vi "Run EU and SR Factories.vi"(8 "error in":errorcluster, 11 "custom device":T1 format="%.0x") -> (0 "error out":errorcluster, 1 "tx execution unit":refnum<class "Tx Execution Unit.lvclass">, 2 "rx execution unit":refnum<class "Rx Execution Unit.lvclass">, 3 "custom device out":T1 format="%.0x", 4 "shared resources":refnum<class "Shared Resources.lvclass">)   [LabVIEW 2020, in "Create Execution Unit.lvclass"]
uses:
  Create Execution Unit.lvclass
  <vilib>/NI VeriStand/Custom Device API/Custom Device Item Ref.ctl
  Engine/Implementation/Tx Execution Unit/Tx Execution Unit.lvclass
  Engine/Implementation/Rx Execution Unit/Rx Execution Unit.lvclass
  Engine/Interfaces/Shared Resources/Shared Resources.lvclass
  Engine/Implementation/Execution Unit Factory/Execution Unit Factory.lvclass
  Engine/Implementation/Shared Resources Factory/Shared Resources Factory.lvclass
  <vilib>/NI VeriStand/Custom Device API/Custom Device API.lvlib
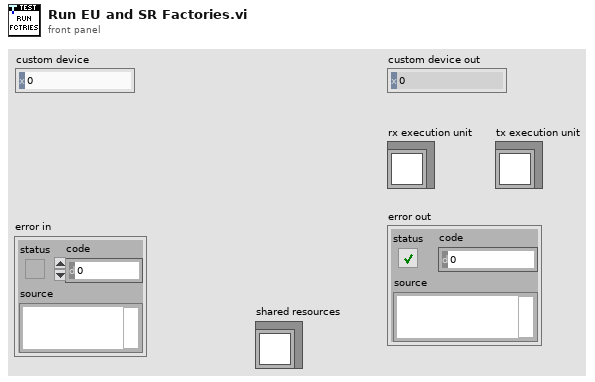
[diagram p1: front panel]
types:
  T1 = typedef "Custom Device API.lvlib/Custom Device Item Ref.ctl" = u64
  T2 = typedef "AIM MIL-STD-1553 Engine.lvlib/Interfaces.lvlib/Execution Unit Information.ctl" = cluster{"Execution Unit":refnum<class "Execution Unit.lvclass">, "Incoming Channels":T1[], "Outgoing Channels":T1[], "ReadWrite Channels":T1[]}
  T3 = cluster{"grouped asynchronous execution units":T2[]}[]
  T4 = cluster{"grouped asynchronous execution units":T2[]}
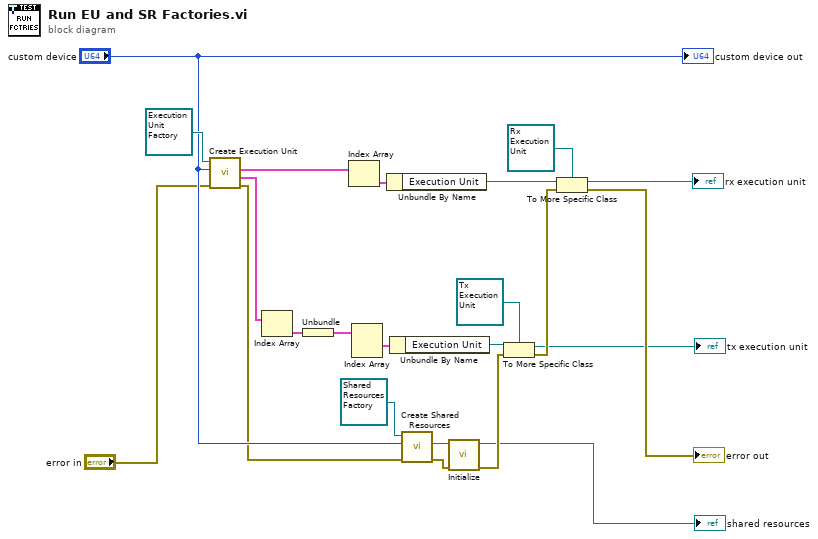
[diagram p0: block diagram]
diagram:
  n1 = call-dynamic "Create Execution Unit.vi"("error in"="error in", "custom device ref"="custom device", "execution unit factory"=refnum<class "Execution Unit Factory.lvclass"> refnum ("Communication Bus Template Interfaces:Implementation.lvlib:Execution Unit Factory.lvclass")) -> ("error out"=w9:errorcluster, "asynchronous execution units"=w23:T3, "inline execution units"=w19:T2[])  [unwired: 5 in, 1 out]
  n2 = Index Array(array=w23) -> (element=w3:T4)  [unwired: 1 in]
  n3 = Unbundle(w3) -> ("grouped asynchronous execution units"=w2:T2[])
  n4 = Index Array(array=w19) -> (element=w20:T2)  [unwired: 1 in]
  n5 = Index Array(array=w2) -> (element #1=w1:T2)  [unwired: 2 in, 1 out]
  n6 = Unbundle By Name(w20) -> ("Execution Unit"=w15:refnum<class "Execution Unit.lvclass">)
  n7 = Unbundle By Name(w1) -> ("Execution Unit"=w16:refnum<class "Execution Unit.lvclass">)
  n8 = call-dynamic "Create Shared Resources.vi"("error in"=w9, "custom device ref"="custom device", "shared resources factory"=refnum<class "Shared Resources Factory.lvclass"> refnum ("Communication Bus Template Interfaces:Implementation.lvlib:Shared Resources Factory.lvclass")) -> ("error out"=w10:errorcluster, "shared resources"=w22:refnum<class "Shared Resources.lvclass">)  [unwired: 6 in, 1 out]
  n9 = call-dynamic "Initialize.vi"("error in"=w10, "shared resources in"=w22) -> ("error out"=w11:errorcluster, "shared resources out"=→"shared resources":refnum<class "Shared Resources.lvclass">)  [unwired: 8 in]
  n10 = To More Specific Class(target class=refnum<class "Tx Execution Unit.lvclass"> refnum ("Communication Bus Template Interfaces:Implementation.lvlib:Tx Execution Unit.lvclass"), reference=w16, error in=w11) -> (specific class reference=→"tx execution unit":refnum<class "Tx Execution Unit.lvclass">, error out=w12:errorcluster)
  n11 = To More Specific Class(target class=refnum<class "Rx Execution Unit.lvclass"> refnum ("Communication Bus Template Interfaces:Implementation.lvlib:Rx Execution Unit.lvclass"), reference=w15, error in=w12) -> (specific class reference=→"rx execution unit":refnum<class "Rx Execution Unit.lvclass">, error out=→"error out":errorcluster)
  "custom device out" <- "custom device"
